vi "SRDG535.ProcCases.vi"(0 "i ref in":refnum<vi>, 1 "selector":string, 2 "Data":T3, 3 "call cluster":T4={"Object"="", "Selector"="", "CallType"=enum."synchronous", "Async Object"="", "Async Selector"="", "Data Descriptor"="", "Data"=[], "Error #"=0, "Expire"=0}, 5 "error in":errorcluster) -> (14 "i ref out":refnum<vi>, 17 "answer cluster":T4={"Object"="", "Selector"="", "CallType"=enum."synchronous", "Async Object"="", "Async Selector"="", "Data Descriptor"="", "Data"=[], "Error #"=0, "Expire"=0}, 19 "error out":errorcluster)   [LabVIEW 2014, in "SRDG535.lvlib"]
doc: "This method is called by a process from within the default case in the event loop. The methods of a class that are linked to events will be called from THIS method. Add your code here."
uses:
  SRDG535.lvlib
  CS_Core/CSSystem/CoreDefs/CoreDefs.call_type.ctl
  CS_Core/BaseProcess/BaseProcess.descriptor string definition.ctl
  CS_Core/CSSystem/CoreDefs/CoreDefs.rawDataType.ctl
  SRDG535.Delay.ctl
  SRDG535.Trigger.ctl
  CS_Core/CSSystem/CoreLib/CoreLib.byte array 2 short.vi
  CS_Core/CSSystem/CoreLib/CoreLib.byte array 2 double.vi
  CS_Core/CSSystem/CoreLib/CoreLib.string 2 byte array.vi
  CS_Core/CSSystem/CoreLib/CoreLib.byte array 2 int.vi
  CS_Core/CSSystem/CoreLib/CoreLib.lvlib
  CS_Core/BaseProcess/BaseProcess.lvlib
  CS_Core/CAEObj/CAEObj.lvlib
  CS_PHELIX/PH_Basics/PH_PSDBWriter/PH_PSDBWriter.lvlib
  CS_PHELIX/PH_Basics/PH_StatusHandler/PH_StatusHandler.lvlib
panel:
  in  "Trigger Settings":T1={"trigger"=0, "Impedance"=FALSE, "Slope"=FALSE, "burst count"=2, "external level (V)"=0.0, "Internal/Burst Rate (Hz)"=0.001, "Burst Period"=4} {"Burst Period" min=4 max=32766; "Internal/Burst Rate (Hz)" min=0.001 max=1000000.0 format="%.3f"; "external level (V)" min=-2.56 max=2.56 format="%.2f"; "burst count" min=2 max=32766; "trigger" scale=0.0..4.0}
  in  "Delay Settings":T2 {"CH D"."Delay (s)" format="%#_13g"; "CH D"."rel to" scale=0.0..3.0; "CH C"."Delay (s)" format="%#_13g"; "CH C"."rel to" scale=0.0..3.0; "CH B"."Delay (s)" format="%#_13g"; "CH B"."rel to" scale=0.0..3.0; "CH A"."Delay (s)" format="%#_13g"; "CH A"."rel to" scale=0.0..3.0}
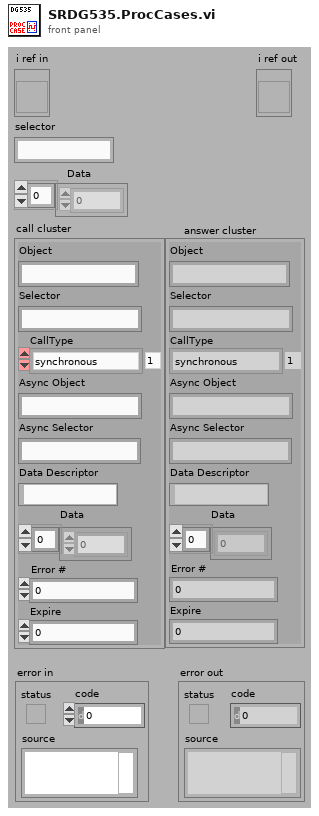
[diagram p1: front panel]
types:
  T1 = typedef "SRDG535.lvlib/SRDG535.Trigger.ctl" = cluster{"trigger":u32, "Impedance":bool, "Slope":bool, "burst count":i32, "external level (V)":sgl, "Internal/Burst Rate (Hz)":dbl, "Burst Period":i32}
  T2 = typedef "SRDG535.lvlib/SRDG535.Delay.ctl" = cluster{"CH A":cluster{"rel to":u32, "Delay (s)":dbl}, "CH B":cluster{"rel to":u32, "Delay (s)":dbl}, "CH C":cluster{"rel to":u32, "Delay (s)":dbl}, "CH D":cluster{"rel to":u32, "Delay (s)":dbl}}
  T3 = typedef "CoreDefs.rawDataType.ctl" = i8[]
  T4 = typedef "CoreDefs.call_type.ctl" = cluster{"Object":string, "Selector":string, "CallType":enum16{"simple", "synchronous", "asynchronous"}, "Async Object":string, "Async Selector":string, "Data Descriptor":T5, "Data":T3, "Error #":i32, "Expire":u32}
  T5 = typedef "BaseProcess.lvlib/BaseProcess.descriptor string definition.ctl" = string
  T6 = typedef "SRDG535.lvlib/SRDG535.i attribute.ctl" = cluster{"GPIB address":string, "Device error":errorcluster, "GUI Refs":cluster{"Delete":refnum<vi>, "Device Error":refnum<vi>, "Information":refnum<vi>, "Output":refnum<vi>, "Delay":refnum<vi>, "Trigger":refnum<vi>}, "Output Settings":T7, "Service ID Rate":i32, "Service IDs Channelinfo":i32[], "Delay Settings":T2, "Trigger Settings":T1}
  T7 = typedef "SRDG535.lvlib/SRDG535.Output.ctl" = cluster{"CH T0":T8, "CH A":T8, "CH B":T8, "CH AB":T8, "CH C":T8, "CH D":T8, "CH CD":T8}
  T8 = typedef "SRDG535.lvlib/SRDG535.Channel Output.ctl" = cluster{"Inversion":bool, "Amplitude (V)":dbl, "Offset (V)":dbl, "Mode":i32, "Load":bool}
  T9 = typedef "PH_PSDBWriter.lvlib/PH_PSDBWriter.PHELIX-Subsystems.ctl" = i32
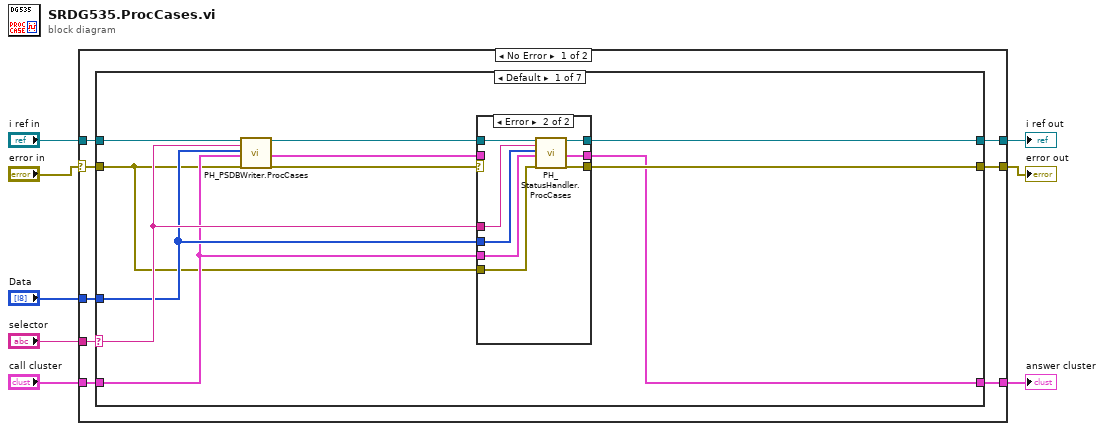
[diagram p0: block diagram]
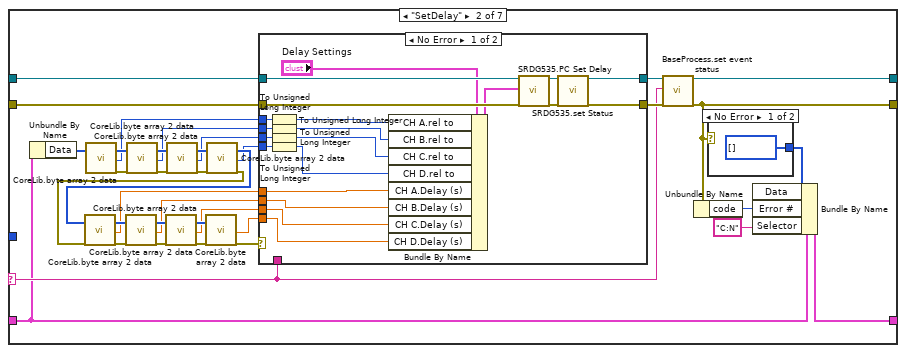
[diagram p3: hidden frame]
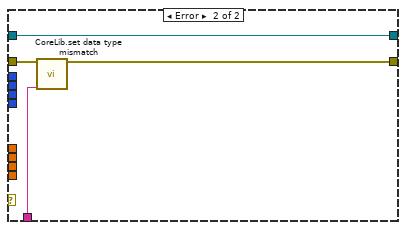
[diagram p4: hidden frame]
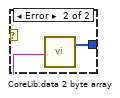
[diagram p5: hidden frame]
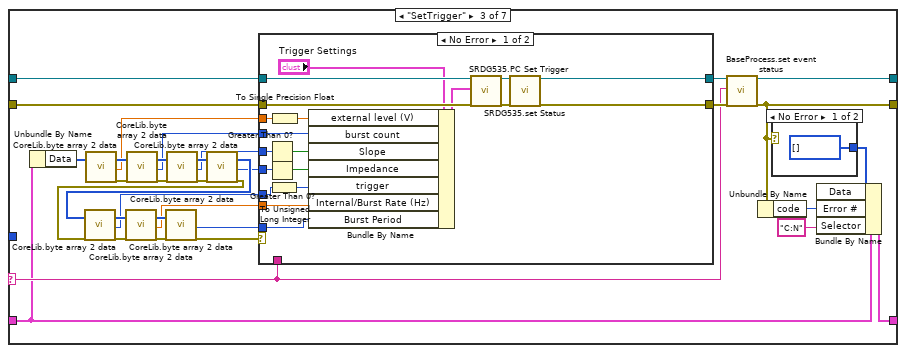
[diagram p6: hidden frame]
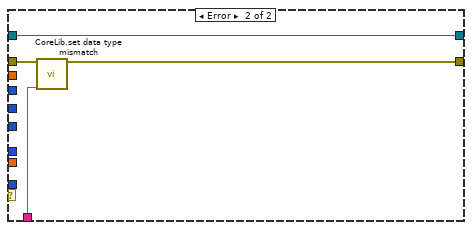
[diagram p7: hidden frame]
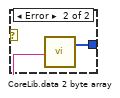
[diagram p8: hidden frame]
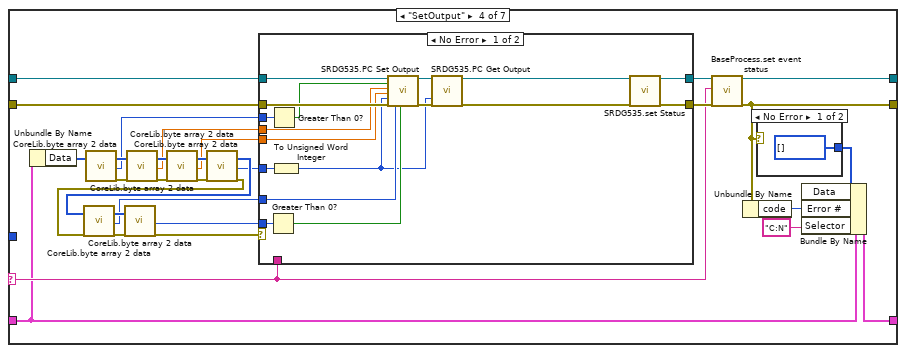
[diagram p9: hidden frame]
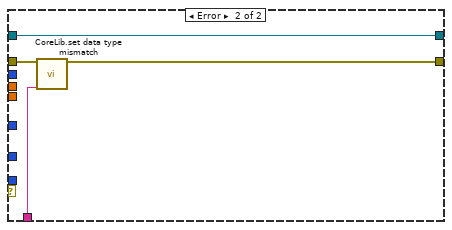
[diagram p10: hidden frame]
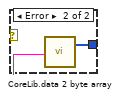
[diagram p11: hidden frame]
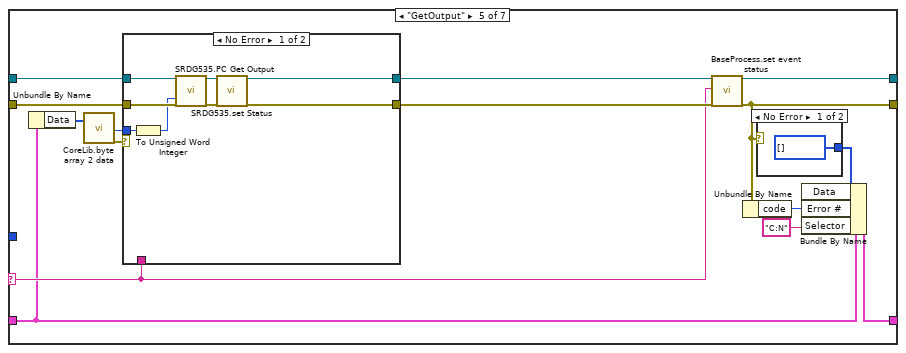
[diagram p12: hidden frame]
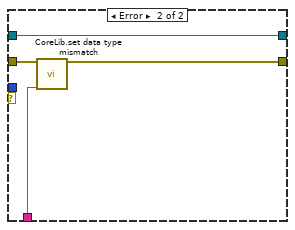
[diagram p13: hidden frame]
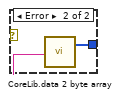
[diagram p14: hidden frame]
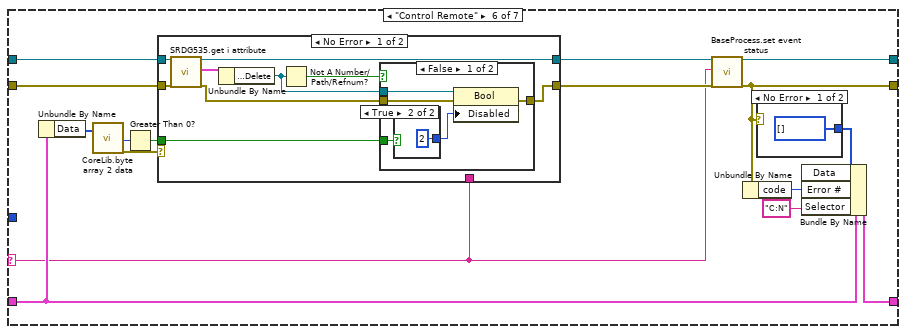
[diagram p15: hidden frame]
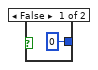
[diagram p16: hidden frame]
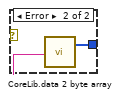
[diagram p19: hidden frame]
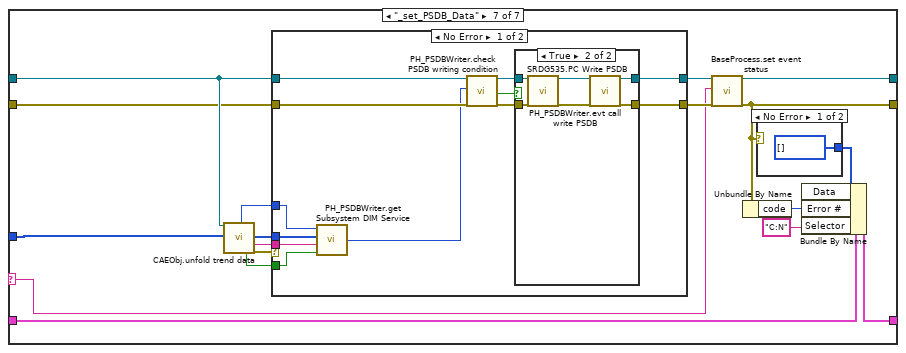
[diagram p20: hidden frame]
diagram:
  n1 = case shown="No Error" "error in" {
    selector: "error in" -> [w9 w334]
    tunnel: "selector" -> [w16 _]
    tunnel: [w15 w335] -> w7
    tunnel: "call cluster" -> [w14 w335]
    tunnel: "i ref in" -> [w13 w336]
    tunnel: [w12 w336] -> w4
    tunnel: [w11 w334] -> w3
    tunnel: "Data" -> [w10 _]
    frame No Error {
      n2 = case shown="Default" w16 {
        selector: w16 -> [w21 w59 w120 w177 w224 w249 w291]
        tunnel: w13 -> [w27 w62 w123 w180 w227 w253 w293]
        tunnel: [w25 w61 w122 w179 w226 w261 w304] -> w12
        tunnel: w14 -> [w19 w57 w118 w175 w222 w250 w301]
        tunnel: [w22 w56 w117 w174 w221 w259 w302] -> w15
        tunnel: w9 -> [w18 w60 w121 w178 w225 w254 w292]
        tunnel: [w23 w58 w119 w176 w223 w260 w303] -> w11
        tunnel: w10 -> [w20 _ _ _ _ _ w290]
        frame Default {
          # "In the default case, always call the ProcCase method of the parent class"
          n3 = call "PH_PSDBWriter.ProcCases.vi"("i ref in"=w27, "selector"=w21, "Data"=w20, "call cluster"=w19, "error in"=w18) -> ("i ref out"=w26:refnum<vi>, "answer cluster"=w17:T4, "error out"=w24:errorcluster)  [unwired: 12 in]
          n4 = case shown="Error" w24 {
            selector: w24 -> [w29 _]
            tunnel: [w29 w38] -> w23
            tunnel: w26 -> [w30 w37]
            tunnel: [w30 w36] -> w25
            tunnel: [w28 w35] -> w22
            tunnel: w18 -> [_ w34]
            tunnel: w19 -> [_ w33]
            tunnel: w20 -> [_ w32]
            tunnel: w21 -> [_ w31]
            tunnel: w17 -> [w28 _]
            frame No Error {
            }
            frame Error {
              n5 = call "PH_StatusHandler.ProcCases.vi"("i ref in"=w37, "selector"=w31, "Data"=w32, "call cluster"=w33, "error in (no error)"=w34) -> ("i ref out"=w36:refnum<vi>, "answer cluster"=w35:T4, "error out"=w38:errorcluster)  [unwired: 12 in]
            }
          }
        }
        frame "SetDelay" {
          n6 = Unbundle By Name(w57) -> ("Data"=w63:T3)
          n7 = call-poly "CoreLib.byte array 2 data.vi"("byteArray"=w63) -> ("byteArray out"=w66:T3, "i16"=w46:i16, "error out"=w69:errorcluster)  [unwired: 16 in]
          n8 = call-poly "CoreLib.byte array 2 data.vi"("byteArray"=w66, "error in (no error)"=w69) -> ("byteArray out"=w65:T3, "i16"=w45:i16, "error out"=w68:errorcluster)  [unwired: 15 in]
          n9 = call-poly "CoreLib.byte array 2 data.vi"("byteArray"=w65, "error in (no error)"=w68) -> ("byteArray out"=w64:T3, "i16"=w44:i16, "error out"=w67:errorcluster)  [unwired: 15 in]
          n10 = call-poly "CoreLib.byte array 2 data.vi"("byteArray"=w64, "error in (no error)"=w67) -> ("byteArray out"=w49:T3, "i16"=w43:i16, "error out"=w48:errorcluster)  [unwired: 15 in]
          n11 = call-poly "CoreLib.byte array 2 data.vi"("byteArray"=w49, "error in (no error)"=w48) -> ("byteArray out"=w52:T3, "d64"=w42:dbl, "error out"=w55:errorcluster)  [unwired: 15 in]
          n12 = call-poly "CoreLib.byte array 2 data.vi"("byteArray"=w52, "error in (no error)"=w55) -> ("byteArray out"=w51:T3, "d64"=w41:dbl, "error out"=w54:errorcluster)  [unwired: 15 in]
          n13 = call-poly "CoreLib.byte array 2 data.vi"("byteArray"=w51, "error in (no error)"=w54) -> ("byteArray out"=w50:T3, "d64"=w40:dbl, "error out"=w53:errorcluster)  [unwired: 15 in]
          n14 = call-poly "CoreLib.byte array 2 data.vi"("byteArray"=w50, "error in (no error)"=w53) -> ("d64"=w39:dbl, "error out"=w47:errorcluster)  [unwired: 15 in, 1 out]
          n15 = case shown="No Error" w47 {
            tunnel: [w87 w98] -> w70
            tunnel: w62 -> [w94 w98]
            tunnel: w60 -> [w93 w97]
            tunnel: [w85 w96] -> w71
            tunnel: w59 -> [_ w95]
            tunnel: w46 -> [w92 _]
            tunnel: w45 -> [w91 _]
            tunnel: w44 -> [w90 _]
            tunnel: w43 -> [w89 _]
            tunnel: w42 -> [w79 _]
            tunnel: w41 -> [w78 _]
            tunnel: w40 -> [w77 _]
            tunnel: w39 -> [w76 _]
            frame No Error {
              n16 = To Unsigned Long Integer(number=w92) -> (unsigned 32bit integer=w83:u32)
              n17 = To Unsigned Long Integer(number=w91) -> (unsigned 32bit integer=w82:u32)
              n18 = To Unsigned Long Integer(number=w90) -> (unsigned 32bit integer=w81:u32)
              n19 = To Unsigned Long Integer(number=w89) -> (unsigned 32bit integer=w80:u32)
              n20 = Bundle By Name(cluster="Delay Settings", "CH A.rel to"=w83, "CH B.rel to"=w82, "CH C.rel to"=w81, "CH D.rel to"=w80, "CH A.Delay (s)"=w79, "CH B.Delay (s)"=w78, "CH C.Delay (s)"=w77, "CH D.Delay (s)"=w76) -> (w75:T2)
              n21 = call "SRDG535.PC Set Delay.vi"("i ref in"=w94, "Delay Settings"=w75, "error IO"=w93) -> ("i ref out"=w88:refnum<vi>, "error out"=w86:errorcluster)  [unwired: 15 in]
              n22 = call "SRDG535.set Status.vi"("i ref in"=w88, "error in"=w86) -> ("i ref out"=w87:refnum<vi>, "error out"=w85:errorcluster)  [unwired: 16 in]
            }
            frame Error {
              n23 = call "CoreLib.set data type mismatch.vi"("error in (no error)"=w97, "error source"=w95) -> ("error out"=w96:errorcluster)  [unwired: 17 in]
            }
          }
          n24 = call "BaseProcess.set event status.vi"("i ref in"=w70, "EventStatus"=w59, "error in (no error)"=w71) -> ("i ref out"=w61:refnum<vi>, "error out"=w58:errorcluster)  [unwired: 14 in, 1 out]
          n25 = Unbundle By Name(w58) -> ("code"=w74:i32)
          n26 = case shown="No Error" w58 {
            selector: w58 -> [_ w102]
            tunnel: [T3 [] ("byteArray out") w100] -> w73
            frame No Error {
            }
            frame Error {
              n27 = Unbundle By Name(w102) -> ("source"=w101:string)
              n28 = call-poly "CoreLib.data 2 byte array.vi"("string"=w101) -> ("byteArray out"=w100:T3)  [unwired: 18 in]
            }
          }
          n29 = Bundle By Name(cluster=w57, "Data"=w73, "Error #"=w74, "Selector"="C:N") -> (w56:T4)
        }
        frame "SetTrigger" {
          n30 = Unbundle By Name(w118) -> ("Data"=w124:T3)
          n31 = call-poly "CoreLib.byte array 2 data.vi"("byteArray"=w124) -> ("byteArray out"=w127:T3, "d64"=w110:dbl, "error out"=w130:errorcluster)  [unwired: 16 in]
          n32 = call-poly "CoreLib.byte array 2 data.vi"("byteArray"=w127, "error in (no error)"=w130) -> ("byteArray out"=w126:T3, "i32"=w109:i32, "error out"=w129:errorcluster)  [unwired: 15 in]
          n33 = call-poly "CoreLib.byte array 2 data.vi"("byteArray"=w126, "error in (no error)"=w129) -> ("byteArray out"=w125:T3, "i16"=w108:i16, "error out"=w128:errorcluster)  [unwired: 15 in]
          n34 = call-poly "CoreLib.byte array 2 data.vi"("byteArray"=w125, "error in (no error)"=w128) -> ("byteArray out"=w112:T3, "i16"=w107:i16, "error out"=w111:errorcluster)  [unwired: 15 in]
          n35 = call-poly "CoreLib.byte array 2 data.vi"("byteArray"=w112, "error in (no error)"=w111) -> ("byteArray out"=w114:T3, "i16"=w106:i16, "error out"=w116:errorcluster)  [unwired: 15 in]
          n36 = call-poly "CoreLib.byte array 2 data.vi"("byteArray"=w114, "error in (no error)"=w116) -> ("byteArray out"=w113:T3, "d64"=w105:dbl, "error out"=w115:errorcluster)  [unwired: 15 in]
          n37 = call-poly "CoreLib.byte array 2 data.vi"("byteArray"=w113, "error in (no error)"=w115) -> ("i32"=w104:i32, "error out"=w103:errorcluster)  [unwired: 15 in, 1 out]
          n38 = case shown="No Error" w103 {
            tunnel: [w146 w158] -> w131
            tunnel: w123 -> [w154 w158]
            tunnel: w121 -> [w153 w157]
            tunnel: [w145 w156] -> w132
            tunnel: w120 -> [_ w155]
            tunnel: w110 -> [w152 _]
            tunnel: w109 -> [w142 _]
            tunnel: w108 -> [w149 _]
            tunnel: w107 -> [w148 _]
            tunnel: w106 -> [w147 _]
            tunnel: w105 -> [w136 _]
            tunnel: w104 -> [w139 _]
            frame No Error {
              n39 = Greater Than 0?(x=w149) -> (x > 0?=w141:bool)
              n40 = Greater Than 0?(x=w148) -> (x > 0?=w140:bool)
              n41 = To Unsigned Long Integer(number=w147) -> (unsigned 32bit integer=w137:u32)
              n42 = To Single Precision Float(number=w152) -> (single precision float=w143:sgl)
              n43 = Bundle By Name(cluster="Trigger Settings", "external level (V)"=w143, "burst count"=w142, "Slope"=w141, "Impedance"=w140, "trigger"=w137, "Internal/Burst Rate (Hz)"=w136, "Burst Period"=w139) -> (w138:T1)
              n44 = call "SRDG535.PC Set Trigger.vi"("i ref in"=w154, "Trigger Settings"=w138, "error IO"=w153) -> ("i ref out"=w151:refnum<vi>, "error out"=w150:errorcluster)  [unwired: 15 in]
              n45 = call "SRDG535.set Status.vi"("i ref in"=w151, "error in"=w150) -> ("i ref out"=w146:refnum<vi>, "error out"=w145:errorcluster)  [unwired: 16 in]
            }
            frame Error {
              n46 = call "CoreLib.set data type mismatch.vi"("error in (no error)"=w157, "error source"=w155) -> ("error out"=w156:errorcluster)  [unwired: 17 in]
            }
          }
          n47 = call "BaseProcess.set event status.vi"("i ref in"=w131, "EventStatus"=w120, "error in (no error)"=w132) -> ("i ref out"=w122:refnum<vi>, "error out"=w119:errorcluster)  [unwired: 14 in, 1 out]
          n48 = Unbundle By Name(w119) -> ("code"=w135:i32)
          n49 = case shown="No Error" w119 {
            selector: w119 -> [_ w162]
            tunnel: [T3 [] ("byteArray out") w160] -> w134
            frame No Error {
            }
            frame Error {
              n50 = Unbundle By Name(w162) -> ("source"=w161:string)
              n51 = call-poly "CoreLib.data 2 byte array.vi"("string"=w161) -> ("byteArray out"=w160:T3)  [unwired: 18 in]
            }
          }
          n52 = Bundle By Name(cluster=w118, "Data"=w134, "Error #"=w135, "Selector"="C:N") -> (w117:T4)
        }
        frame "SetOutput" {
          n53 = Unbundle By Name(w175) -> ("Data"=w181:T3)
          n54 = call-poly "CoreLib.byte array 2 data.vi"("byteArray"=w181) -> ("byteArray out"=w184:T3, "i16"=w169:i16, "error out"=w187:errorcluster)  [unwired: 16 in]
          n55 = call-poly "CoreLib.byte array 2 data.vi"("byteArray"=w184, "error in (no error)"=w187) -> ("byteArray out"=w183:T3, "d64"=w168:dbl, "error out"=w186:errorcluster)  [unwired: 15 in]
          n56 = call-poly "CoreLib.byte array 2 data.vi"("byteArray"=w183, "error in (no error)"=w186) -> ("byteArray out"=w182:T3, "d64"=w167:dbl, "error out"=w185:errorcluster)  [unwired: 15 in]
          n57 = call-poly "CoreLib.byte array 2 data.vi"("byteArray"=w182, "error in (no error)"=w185) -> ("byteArray out"=w171:T3, "i16"=w166:i16, "error out"=w170:errorcluster)  [unwired: 15 in]
          n58 = call-poly "CoreLib.byte array 2 data.vi"("byteArray"=w171, "error in (no error)"=w170) -> ("byteArray out"=w172:T3, "i32"=w165:i32, "error out"=w173:errorcluster)  [unwired: 15 in]
          n59 = call-poly "CoreLib.byte array 2 data.vi"("byteArray"=w172, "error in (no error)"=w173) -> ("i16"=w164:i16, "error out"=w163:errorcluster)  [unwired: 15 in, 1 out]
          n60 = case shown="No Error" w163 {
            tunnel: [w207 w213] -> w188
            tunnel: w180 -> [w209 w213]
            tunnel: w178 -> [w208 w212]
            tunnel: [w198 w211] -> w189
            tunnel: w177 -> [_ w210]
            tunnel: w169 -> [w206 _]
            tunnel: w168 -> [w204 _]
            tunnel: w167 -> [w203 _]
            tunnel: w166 -> [w202 _]
            tunnel: w165 -> [w201 _]
            tunnel: w164 -> [w200 _]
            frame No Error {
              n61 = Greater Than 0?(x=w200) -> (x > 0?=w199:bool)
              n62 = Greater Than 0?(x=w206) -> (x > 0?=w205:bool)
              n63 = To Unsigned Word Integer(number=w202) -> (unsigned 16bit integer=w193:u16)
              n64 = call "SRDG535.PC Set Output.vi"("i ref in"=w209, "inversion"=w205, "amplitude"=w204, "offset"=w203, "output"=w193, "error IO"=w208, "mode"=w201, "load"=w199) -> ("i ref out"=w197:refnum<vi>, "error out"=w195:errorcluster)  [unwired: 10 in]
              n65 = call "SRDG535.PC Get Output.vi"("i ref in"=w197, "Channel"=w193, "error IO"=w195) -> ("i ref out"=w196:refnum<vi>, "error out"=w194:errorcluster)  [unwired: 15 in]
              n66 = call "SRDG535.set Status.vi"("i ref in"=w196, "error in"=w194) -> ("i ref out"=w207:refnum<vi>, "error out"=w198:errorcluster)  [unwired: 16 in]
            }
            frame Error {
              n67 = call "CoreLib.set data type mismatch.vi"("error in (no error)"=w212, "error source"=w210) -> ("error out"=w211:errorcluster)  [unwired: 17 in]
            }
          }
          n68 = call "BaseProcess.set event status.vi"("i ref in"=w188, "EventStatus"=w177, "error in (no error)"=w189) -> ("i ref out"=w179:refnum<vi>, "error out"=w176:errorcluster)  [unwired: 14 in, 1 out]
          n69 = Unbundle By Name(w176) -> ("code"=w192:i32)
          n70 = case shown="No Error" w176 {
            selector: w176 -> [_ w217]
            tunnel: [T3 [] ("byteArray out") w215] -> w191
            frame No Error {
            }
            frame Error {
              n71 = Unbundle By Name(w217) -> ("source"=w216:string)
              n72 = call-poly "CoreLib.data 2 byte array.vi"("string"=w216) -> ("byteArray out"=w215:T3)  [unwired: 18 in]
            }
          }
          n73 = Bundle By Name(cluster=w175, "Data"=w191, "Error #"=w192, "Selector"="C:N") -> (w174:T4)
        }
        frame "GetOutput" {
          n74 = Unbundle By Name(w222) -> ("Data"=w219:T3)
          n75 = call-poly "CoreLib.byte array 2 data.vi"("byteArray"=w219) -> ("i16"=w220:i16, "error out"=w218:errorcluster)  [unwired: 16 in, 1 out]
          n76 = case shown="No Error" w218 {
            tunnel: [w235 w244] -> w228
            tunnel: w227 -> [w240 w244]
            tunnel: w225 -> [w239 w243]
            tunnel: [w233 w242] -> w229
            tunnel: w224 -> [_ w241]
            tunnel: w220 -> [w238 _]
            frame No Error {
              n77 = To Unsigned Word Integer(number=w238) -> (unsigned 16bit integer=w237:u16)
              n78 = call "SRDG535.PC Get Output.vi"("i ref in"=w240, "Channel"=w237, "error IO"=w239) -> ("i ref out"=w236:refnum<vi>, "error out"=w234:errorcluster)  [unwired: 15 in]
              n79 = call "SRDG535.set Status.vi"("i ref in"=w236, "error in"=w234) -> ("i ref out"=w235:refnum<vi>, "error out"=w233:errorcluster)  [unwired: 16 in]
            }
            frame Error {
              n80 = call "CoreLib.set data type mismatch.vi"("error in (no error)"=w243, "error source"=w241) -> ("error out"=w242:errorcluster)  [unwired: 17 in]
            }
          }
          n81 = call "BaseProcess.set event status.vi"("i ref in"=w228, "EventStatus"=w224, "error in (no error)"=w229) -> ("i ref out"=w226:refnum<vi>, "error out"=w223:errorcluster)  [unwired: 14 in, 1 out]
          n82 = Unbundle By Name(w223) -> ("code"=w232:i32)
          n83 = case shown="No Error" w223 {
            selector: w223 -> [_ w248]
            tunnel: [T3 [] ("byteArray out") w246] -> w231
            frame No Error {
            }
            frame Error {
              n84 = Unbundle By Name(w248) -> ("source"=w247:string)
              n85 = call-poly "CoreLib.data 2 byte array.vi"("string"=w247) -> ("byteArray out"=w246:T3)  [unwired: 18 in]
            }
          }
          n86 = Bundle By Name(cluster=w222, "Data"=w231, "Error #"=w232, "Selector"="C:N") -> (w221:T4)
        }
        frame "Control Remote" {
          n87 = Unbundle By Name(w250) -> ("Data"=w255:T3)
          n88 = call-poly "CoreLib.byte array 2 data.vi"("byteArray"=w255) -> ("i16"=w256:i16, "error out"=w258:errorcluster)  [unwired: 16 in, 1 out]
          n89 = Greater Than 0?(x=w256) -> (x > 0?=w257:bool)
          n90 = case shown="No Error" w258 {
            tunnel: [w267 w285] -> w252
            tunnel: w253 -> [w273 w285]
            tunnel: w254 -> [w272 w284]
            tunnel: [w268 w283] -> w251
            tunnel: w249 -> [_ w282]
            tunnel: w257 -> [w269 _]
            frame No Error {
              n91 = call "SRDG535.get i attribute.vi"("i ref in"=w273, "error in (no error)"=w272) -> ("i ref out"=w267:refnum<vi>, "i attribute"=w271:T6, "error out"=w270:errorcluster)  [unwired: 15 in]
              n92 = Unbundle By Name(w271) -> ("GUI Refs.Delete"=w266:refnum<vi>)
              n93 = Not A Number/Path/Refnum?(number/path/refnum=w266) -> (NaN/Path/Refnum?=w265:bool)
              n94 = case shown="False" w265 {
                tunnel: w266 -> [w278 _]
                tunnel: w270 -> [w277 w281]
                tunnel: [w276 w281] -> w268
                tunnel: w269 -> [w275 _]
                frame False {
                  n95 = case shown="True" w275 {
                    tunnel: [0 2] -> w274
                    frame False {
                    }
                    frame True {
                    }
                  }
                  n96 = property class="Bool"(reference=w278, error in=w277, "Disabled"=w274) -> (error out=w276:errorcluster)  [unwired: 1 out]
                }
                frame True {
                }
              }
            }
            frame Error {
              n97 = call "CoreLib.set data type mismatch.vi"("error in (no error)"=w284, "error source"=w282) -> ("error out"=w283:errorcluster)  [unwired: 17 in]
            }
          }
          n98 = call "BaseProcess.set event status.vi"("i ref in"=w252, "EventStatus"=w249, "error in (no error)"=w251) -> ("i ref out"=w261:refnum<vi>, "error out"=w260:errorcluster)  [unwired: 14 in, 1 out]
          n99 = Unbundle By Name(w260) -> ("code"=w264:i32)
          n100 = case shown="No Error" w260 {
            selector: w260 -> [_ w289]
            tunnel: [T3 [] ("byteArray out") w287] -> w263
            frame No Error {
            }
            frame Error {
              n101 = Unbundle By Name(w289) -> ("source"=w288:string)
              n102 = call-poly "CoreLib.data 2 byte array.vi"("string"=w288) -> ("byteArray out"=w287:T3)  [unwired: 18 in]
            }
          }
          n103 = Bundle By Name(cluster=w250, "Data"=w263, "Error #"=w264, "Selector"="C:N") -> (w259:T4)
        }
        frame "_set_PSDB_Data" {
          n104 = call "CAEObj.unfold trend data.vi"("i ref in"=w293, "raw trend data"=w290) -> ("quality"=w296:i32, "no link"=w299:bool, "data"=w297:i8[], "typeDescriptor"=w298:string, "error out"=w300:errorcluster)  [unwired: 9 in, 4 out]
          n105 = case shown="No Error" w300 {
            tunnel: w292 -> [w319 w329]
            tunnel: [w318 w328] -> w295
            tunnel: [w317 w329] -> w294
            tunnel: w293 -> [w315 w328]
            tunnel: w299 -> [w308 _]
            tunnel: w298 -> [w310 _]
            tunnel: w297 -> [w311 _]
            tunnel: w296 -> [w309 _]
            frame No Error {
              n106 = call "PH_PSDBWriter.get Subsystem DIM Service.vi"("no link"=w308, "typeDescriptor"=w310, "data"=w311, "quality"=w309) -> ("PHELIX Subsystems"=w312:T9)
              n107 = call "PH_PSDBWriter.check PSDB writing condition.vi"("i ref in"=w315, "wanted Subsystem"=w312, "error IO"=w319) -> ("i ref out"=w314:refnum<vi>, "write PSDB?"=w313:bool, "error out"=w316:errorcluster)  [unwired: 14 in]
              n108 = case shown="True" w313 {
                tunnel: w316 -> [w320 w327]
                tunnel: [w321 w324] -> w318
                tunnel: [w320 w322] -> w317
                tunnel: w314 -> [w321 w326]
                frame False {
                }
                frame True {
                  n109 = call "SRDG535.PC Write PSDB.vi"("i ref in"=w326, "error IO"=w327) -> ("i ref out"=w325:refnum<vi>, "error out"=w323:errorcluster)  [unwired: 16 in]
                  n110 = call "PH_PSDBWriter.evt call write PSDB.vi"("i ref in"=w325, "error in (no error)"=w323) -> ("i ref out"=w324:refnum<vi>, "error out"=w322:errorcluster)  [unwired: 16 in]
                }
              }
            }
            frame Error {
            }
          }
          n111 = call "BaseProcess.set event status.vi"("i ref in"=w295, "EventStatus"=w291, "error in (no error)"=w294) -> ("i ref out"=w304:refnum<vi>, "error out"=w303:errorcluster)  [unwired: 14 in, 1 out]
          n112 = Unbundle By Name(w303) -> ("code"=w307:i32)
          n113 = case shown="No Error" w303 {
            selector: w303 -> [_ w333]
            tunnel: [T3 [] ("byteArray out") w331] -> w306
            frame No Error {
            }
            frame Error {
              n114 = Unbundle By Name(w333) -> ("source"=w332:string)
              n115 = call-poly "CoreLib.data 2 byte array.vi"("string"=w332) -> ("byteArray out"=w331:T3)  [unwired: 18 in]
            }
          }
          n116 = Bundle By Name(cluster=w301, "Data"=w306, "Error #"=w307, "Selector"="C:N") -> (w302:T4)
        }
      }
    }
    frame Error {
    }
  }
  "answer cluster" <- w7
  "i ref out" <- w4
  "error out" <- w3
